vi "RegisterMap_ADSxxxx.vi"(8 "error in (no error)":errorcluster, 11 "Register Map File":path) -> (0 "error out":errorcluster, 2 "Register Names":string[](array[string]), 3 "ADSxxxx Register Data":T1[](array[typedef]) {"Base" format="%.0x"; "Item Count" format="%.0x"; "Value" format="%.0x"; "RegMap"."Mask" format="%.0x"; "Default" format="%.0x"; "Register" format="%.0x"})   [LabVIEW 2010]
doc: "This VI loads the information from the register map text file into an array to be used as a shadow register.\nThis VI can also be used to create/update the register enum used in the top-level VI.\n\nInputs:\nRegister Map File - (path) path and file name of the register map text file (see subVIs for format).\nRegsister Enum - (path) path to the typdef enum to update with the register names (if enabled)\nCreate Enum? - (bool) TRUE will create/update an enum specified in Register Enum\nerror in - error input cluster\n\nOutputs:\nAMC7812 Register Data - (cluster[]) array of clusters containing the information from the text file\nRegister Names - (str[]) string array containing the register names to be used to index register by name.\nerror out - error output cluster"
uses:
  TYP_ADSxxxx Register.ctl
  TYP_RegMap Item.ctl
panel:
  in  "Create Enum?":bool
  in  "Register Enum":path
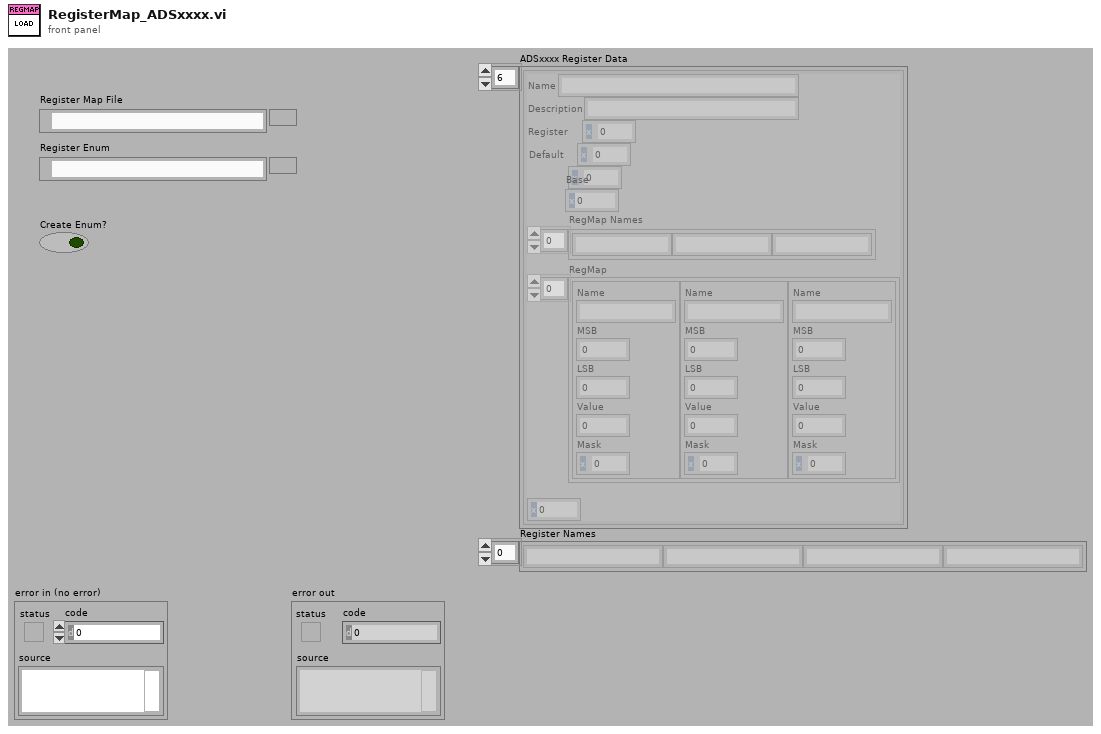
[diagram p1: front panel]
types:
  T1 = typedef "TYP_ADSxxxx Register.ctl" = cluster{"Name":string, "Description":string, "Register":u16, "Default":u16, "Value":u16, "Base":u16, "RegMap Names":string[], "RegMap":T2[], "Item Count":u8}
  T2 = typedef "TYP_RegMap Item.ctl" = cluster{"Name":string, "MSB":u16, "LSB":u16, "Value":u16, "Mask":u16}
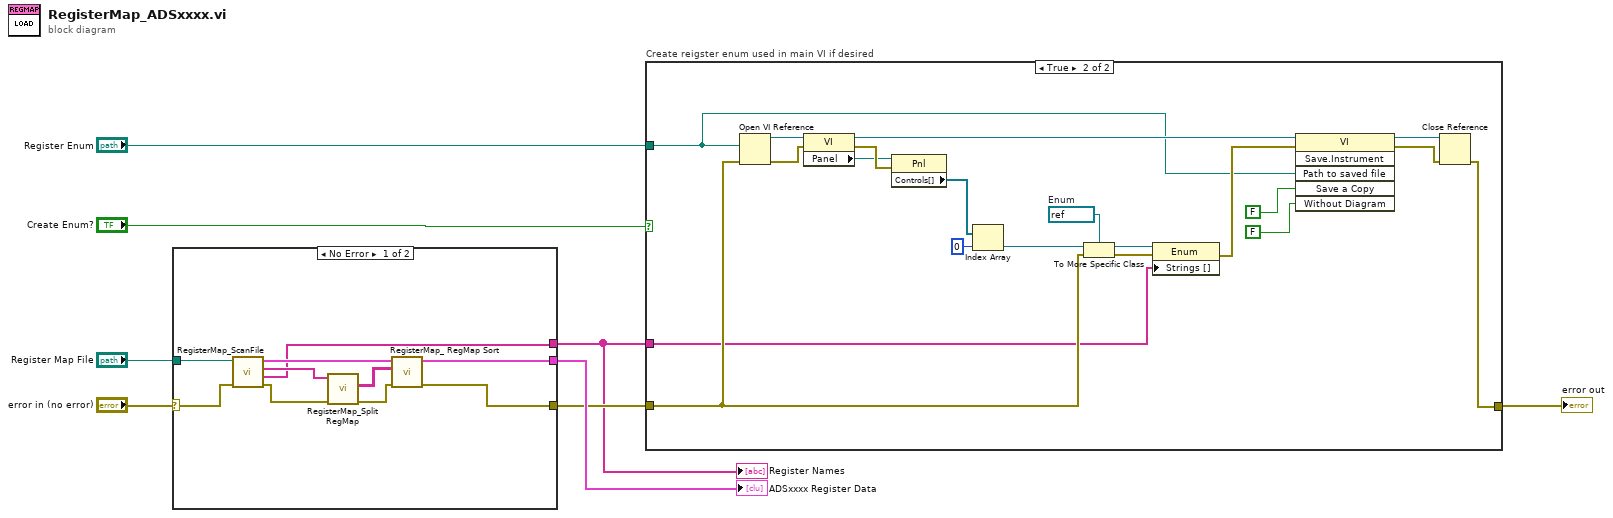
[diagram p0: block diagram]
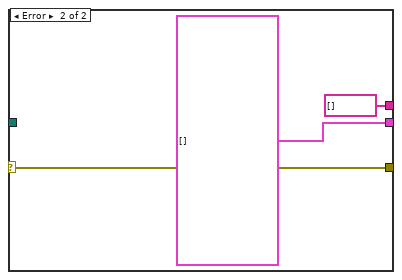
[diagram p3: hidden frame]
diagram:
  n1 = case shown="No Error" "error in (no error)" {
    selector: "error in (no error)" -> [w12 w21]
    tunnel: "Register Map File" -> [w18 _]
    tunnel: [w11 w21] -> w5
    tunnel: [w10 T1[] [] ("Registers Output")] -> w6
    tunnel: [w9 string[] [] ("Register Names")] -> w2
    frame No Error {
      n2 = call "RegisterMap_ScanFile.vi"("error in (no error)"=w12, "Register Map File"=w18) -> ("error out"=w14:errorcluster, "Register Names"=w9:string[], "Register RegMap Data"=w17:string[], "ADC Registers"=w16:T1[])  [unwired: 6 out]
      n3 = call "RegisterMap_Split RegMap.vi"("error in (no error)"=w14, "Register RegMap Strings"=w17) -> ("error out"=w13:errorcluster, "Register RegMap Data"=w15:string[][])  [unwired: 8 out]
      n4 = call "RegisterMap_ RegMap Sort.vi"("error in (no error)"=w13, "Register RegMap Data"=w15, "Register Data IN"=w16) -> ("error out"=w11:errorcluster, "Register Data OUT"=w10:T1[])  [unwired: 7 out]
    }
    frame Error {
    }
  }
  "ADSxxxx Register Data" <- w6
  "Register Names" <- w2
  n5 = case "Create reigster enum used in main VI if desired" shown="True" "Create Enum?" {
    tunnel: w5 -> [w22 w26]
    tunnel: "Register Enum" -> [_ w24]
    tunnel: w2 -> [_ w25]
    tunnel: [w22 w23] -> w1
    frame False {
    }
    frame True {
      w37 = refnum<vi> refnum  # Enum
      n6 = Open VI Reference(vi path=w24, error in (no error)=w26) -> (vi reference=w30:refnum<vi>, error out=w28:errorcluster)  [unwired: 2 in, 2 out]
      n7 = property class="VI"(reference=w30, error in=w28) -> (reference out=w29:refnum<vi>, error out=w42:errorcluster, "Panel"=w41:refnum<vi>)
      n8 = property class="Pnl"(reference=w41, error in=w42) -> ("Controls[]"=w40:refnum<vi>[])  [unwired: 2 out]
      n9 = Index Array(array=w40, index=0) -> (element=w38:refnum<vi>)
      n10 = To More Specific Class(target class=w37, reference=w38, error in=w26) -> (specific class reference=w32:refnum<vi>, error out=w27:errorcluster)
      n11 = property class="Enum"(reference=w32, error in=w27, "Strings []"=w25) -> (error out=w31:errorcluster)  [unwired: 1 out]
      n12 = invoke class="VI" method="Save.Instrument"(reference=w29, error in=w31, "Path to saved file"=w24, "Save a Copy"=FALSE, "Without Diagram"=FALSE) -> (reference out=w34:refnum<vi>, error out=w33:errorcluster)  [unwired: 1 in, 4 out]
      n13 = Close Reference(reference=w34, error in (no error)=w33) -> (error out=w23:errorcluster)
    }
  }
  "error out" <- w1
